vi "Set Trigger Source.vi"(7 "Action (Default: Set and Validate)":T1, 8 "error in (no error)":errorcluster, 10 "Source":string, 11 "Camera in":refnum<class "Camera.lvclass">) -> (0 "error out":errorcluster, 3 "Camera":refnum<class "Camera.lvclass">)   [LabVIEW 2020, in "Camera.lvclass"]
uses:
  Camera.lvclass
  Value Set Action.ctl
  Camera.lvclass/Camera.ctl
  bin/gindustrialcam_32-1.dll
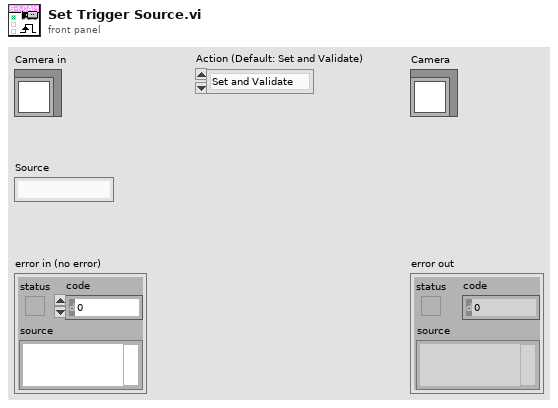
[diagram p1: front panel]
types:
  T1 = typedef "Camera.lvclass/Value Set Action.ctl" = enum16{"Set and Validate", "Set Only"}
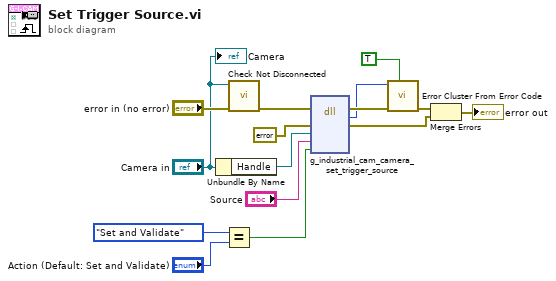
[diagram p0: block diagram]
diagram:
  n1 = Unbundle By Name("Camera in") -> ("Handle"=w7:refnum<data-value>)
  n2 = Equal?(x=Value_Set_Action."Set and Validate" ("Valye Set Action"), y="Action (Default: Set and Validate)") -> (x = y?=w2:bool)
  n3 = call "Check Not Disconnected.vi"("error in (no error)"="error in (no error)", "Camera in"="Camera in") -> ("error out"=w6:errorcluster)  [unwired: 9 in]
  n4 = dll-call lib="C:/Workspace/SSDC/g-industrial-camera/LabVIEW/g_industrial_cam/bin/gindustrialcam_*-1.*" fn="g_industrial_cam_camera_set_trigger_source"(error in=w6, "err"=errorcluster {"status"=FALSE, "code"=0, "source"=""} ("error constant"), "edvr"=w7, "source"="Source", "set_and_validate"=w2) -> (error out=w13:errorcluster, "Mg_Error"=w12:i32, "err"=w10:errorcluster)  [unwired: 5 in, 1 out]
  n5 = call <vilib>:"Error Cluster From Error Code.vi"("show call chain? (False)"=TRUE, "error in (no error)"=w13, "error code (0)"=w12) -> ("error out"=w11:errorcluster)  [unwired: 6 in]
  n6 = Merge Errors(w11, w10) -> (→"error out":errorcluster)
  "Camera" <- "Camera in"
